vi "Populate Device Info.vi"(8 "error in":errorcluster, 11 "UI Actor in":refnum<class "UI Actor.lvclass">) -> (0 "error out":errorcluster)   [LabVIEW 2019, in "UI Actor.lvlib" / "UI Actor.lvclass"]
uses:
  UI Actor.lvclass
  UI Actor.lvclass/UI Actor.ctl
  Controls/Device Info.ctl
  UI Actor.lvlib
  Electronic Datasheet/Electronic Datasheet.lvclass
  Core/Device Info/Device Info.lvclass
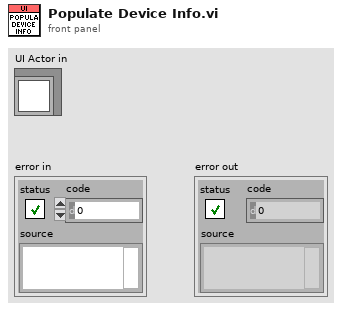
[diagram p1: front panel]
types:
  T1 = typedef "UI Actor.lvlib/Device Info.ctl" = cluster{"ProductName":string, "ProductNumber":u32, "VendorName":string, "VendorNumber":u32}
  T2 = map{path, refnum<class "Electronic Datasheet.lvclass">}
  T3 = cluster{"VendorName":string, "VendorNumber":u32, "ProductName":string, "ProductNumber":u32, "RevisionNumber":u32, "OrderCode":string, "BaudRate_10":bool, "BaudRate_20":bool, "BaudRate_50":bool, "BaudRate_125":bool, "BaudRate_250":bool, "BaudRate_500":bool, "BaudRate_800":bool, "BaudRate_1000":bool, "BaudRate_auto":bool, "SimpleBootUpMaster":bool, "SimpleBootUpSlave":bool, "Granularity":u8, "DynamicChannelsSupported":bool, "CompactPDO":u8, "GroupMessaging":bool, "NrOfRXPDO":u16, "NrOfTXPDO":u16, "LSS_Supported":bool, "LSS_Master":bool, "NG_Slave":bool, "NG_Master":bool, "NrOfNG_MonitoredNodes":u16}
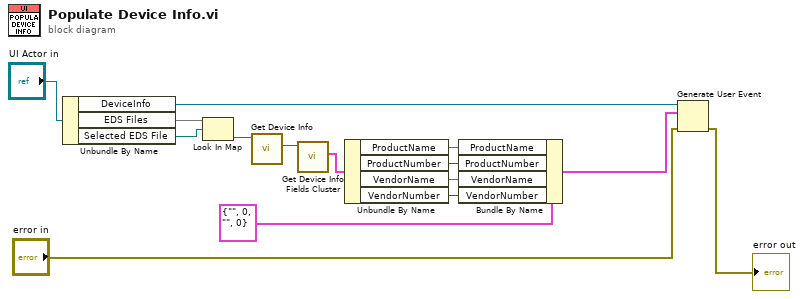
[diagram p0: block diagram]
diagram:
  n1 = Unbundle By Name("UI Actor in") -> ("DeviceInfo"=w14:refnum<user-event>, "EDS Files"=w12:T2, "Selected EDS File"=w10:path)
  n2 = Look In Map(map=w12, key=w10) -> (value=w11:refnum<class "Electronic Datasheet.lvclass">)  [unwired: 1 in, 1 out]
  n3 = call "Get Device Info.vi"("reference in"=w11) -> ("Device Info"=w9:refnum<class "Device Info.lvclass">)  [unwired: 8 in, 2 out]
  n4 = call "Get Device Info Fields Cluster.vi"("Device Info in"=w9) -> ("Device Info"=w7:T3)  [unwired: 9 in, 1 out]
  n5 = Unbundle By Name(w7) -> ("ProductName"=w1:string, "ProductNumber"=w2:u32, "VendorName"=w3:string, "VendorNumber"=w4:u32)
  n6 = Bundle By Name(cluster=T1 {"ProductName"="", "ProductNumber"=0, "VendorName"="", "VendorNumber"=0} ("DeviceInfo"), "ProductName"=w1, "ProductNumber"=w2, "VendorName"=w3, "VendorNumber"=w4) -> (w5:T1)
  n7 = Generate User Event(user event=w14, event data cluster=w5, error in="error in") -> (error out=→"error out":errorcluster)  [unwired: 1 in, 1 out]
